vi "Wait For LACK OF Front Panel Activity (event driven).vi"(0 "Front Panel to Monitor (calling VI)":refnum<vi>, 1 "Minimum Wait Time (ms)":i32=1000) -> (8 "Actual Wait Time (ms)":i64)   [LabVIEW 2013, in "FindName Task_Manager.lvlib"]
doc: "Pauses execution of the calling VI block diagram, until the function detects A LACK OF front panel activity for the specified contiguous wait time, in the front panel being monitored. By default, the front pannel to be monitored is that of the VI calling this function, but this can be specified to be any other VI for which you have a reference to. The actual measured wait time is returned. If \"Front Panel to Monitor\" is unwired or is otherwise not a valid reference, then the calling VI will be monitored. If the calling VI ALSO has an invalid reference, then this function will return immediately, and \"actual wait time\" will be -1.\n\nThis variation is event driven, allowing for more flexibility in what constitutes front pannel \"activity\". For example, the non-event driven variation of this VI does not consider mouse movement across the front panel as activity, but this variation can do so."
uses:
  FindName Task_Manager.lvlib
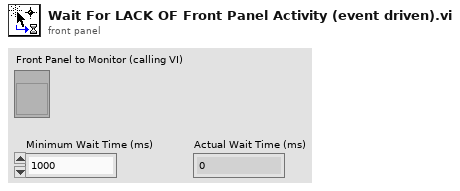
[diagram p1: front panel]
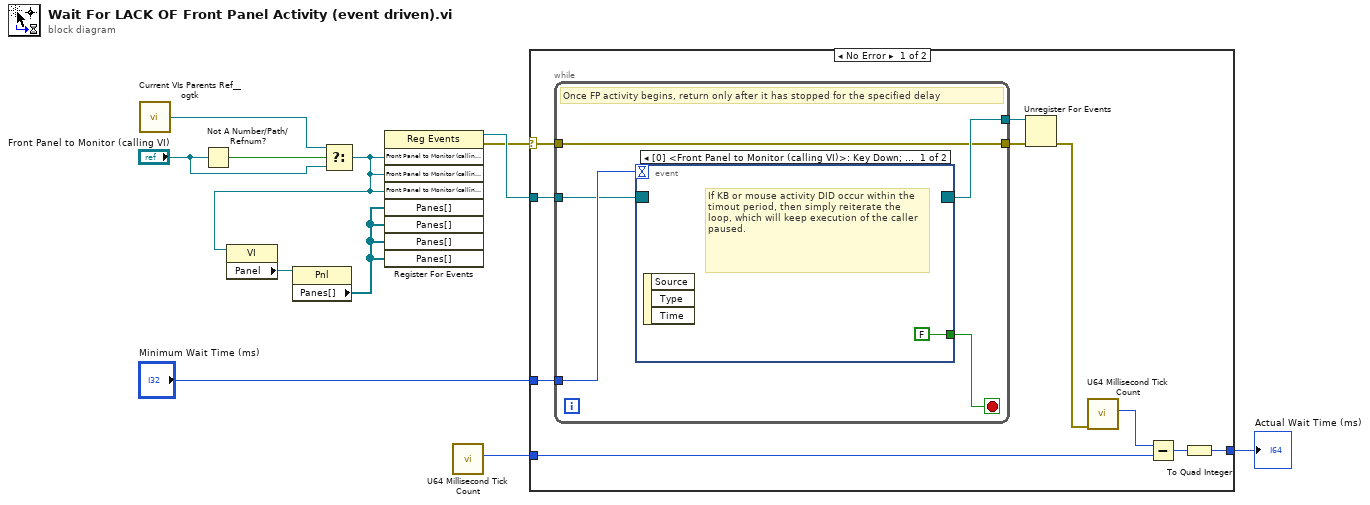
[diagram p0: block diagram]
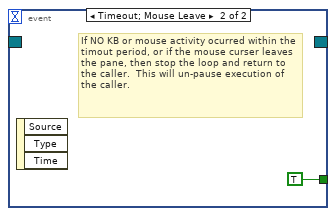
[diagram p2: hidden frame]
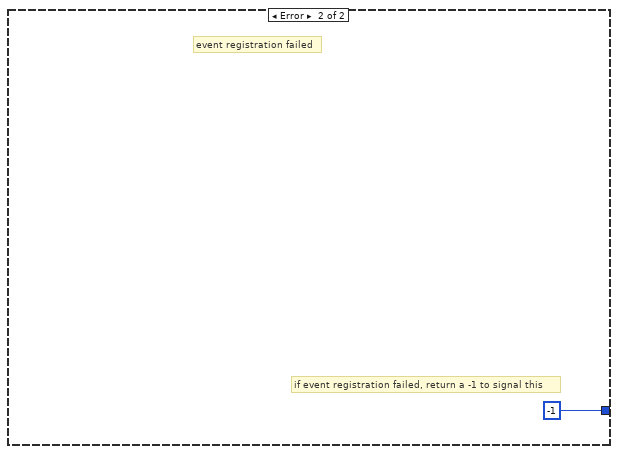
[diagram p3: hidden frame]
diagram:
  n1 = call "Current VIs Parents Ref__ogtk.vi"() -> ("Calling VI's Reference"=w4:refnum<vi>)  [unwired: 2 in]
  n2 = Not A Number/Path/Refnum?(number/path/refnum="Front Panel to Monitor (calling VI)") -> (NaN/Path/Refnum?=w6:bool)
  n3 = Select(t=w4, s=w6, f="Front Panel to Monitor (calling VI)") -> (s? t:f=w1:refnum<vi>)
  n4 = property class="VI"(reference=w1) -> ("Panel"=w3:refnum<vi>)  [unwired: 1 in, 2 out]
  n5 = property class="Pnl"(reference=w3) -> ("Panes[]"=w2:refnum<vi>[])  [unwired: 1 in, 2 out]
  n6 = register-events(w1, w1, w1, w2, w2, w2, w2) -> (reference out=w10:refnum<event-registration>, error out=w9:errorcluster)  [unwired: 2 in]
  n7 = call "U64 Millisecond Tick Count.vi"() -> ("U64 millisecond \ntimer value"=w8:u64)  [unwired: 10 in, 1 out]
  n8 = case shown="No Error" w9 {
    selector: w9 -> [w17 _]
    tunnel: "Minimum Wait Time (ms)" -> [w21 _]
    tunnel: w10 -> [w20 _]
    tunnel: w8 -> [w15 _]
    tunnel: [w14 i64 -1] -> w7
    frame No Error {
      n9 = while {
        tunnel: w21 -> [w26]
        tunnel: w20 -> [w24]
        tunnel: [w23] -> w19
        tunnel: w17 -> [w22]
        tunnel: [w22] -> w18
        stop <- w25 stop-if-true
        # "Once FP activity begins, return only after it has stopped for the specified delay"
        n10 = event shown="[0] <Front Panel to Monitor (calling VI)>: Key Down;  <Front Panel to Monitor (calling VI)>: Key Up;  <Front Panel to Monitor (calling VI)>: Key Repeat;  <Panes[]>: Mouse Down;  <Panes[]>: Mouse Up;  <Panes[]>: Mouse Move" {
          selector: w24 -> [_ _]
          dyn-events: [_ _] -> w23
          timeout: w26 -> [_ _]
          tunnel: [FALSE TRUE] -> w25
          event Key Down; Key Up; Key Repeat; Mouse Down; Mouse Up; Mouse Move {
            # "If KB or mouse activity DID occur within the timout period, then simply reiterate the loop, which will keep execution of the caller paused."
            n11 = event-data() -> ()  [unwired: 1 in, 3 out]
          }
          event Timeout; Mouse Leave {
            # "If NO KB or mouse activity ocurred within the timout period, or if the mouse curser leaves the pane, then stop the loop and return to the caller.  This will un-pause execution of the caller."
            n12 = event-data() -> ()  [unwired: 1 in, 3 out]
          }
        }
      }
      n13 = Unregister For Events(event registration refnum=w19, error in=w18) -> (error out=w12:errorcluster)
      n14 = call "U64 Millisecond Tick Count.vi"("Error In"=w12) -> ("U64 millisecond \ntimer value"=w13:u64)  [unwired: 9 in, 1 out]
      n15 = Subtract(x=w13, y=w15) -> (x-y=w16:u64)
      n16 = To Quad Integer(1:w16) -> (0:w14:i64)
    }
    frame Error {
      # "if event registration failed, return a -1 to signal this"
      # "event registration failed"
    }
  }
  "Actual Wait Time (ms)" <- w7
